vi "Delete Messages.vi"(8 "error in (no error)":errorcluster, 10 "Message":variant, 11 "Telegram Class in":refnum<class "Telegram Class.lvclass">) -> (0 "error out":errorcluster, 3 "Telegram Class out":refnum<class "Telegram Class.lvclass">)   [LabVIEW 2015, in "Telegram Library.lvlib" / "Telegram Class.lvclass"]
doc: "Created IvanLis by LabVIEW Portal\nProfile: http://labviewportal.org/memberlist.php?mode=viewprofile&u=987\neMail: IvanLisanov@gMail.com\nTelegram: https://t.me/IvanLis"
uses:
  Telegram Class.lvclass
  JSON Library/TypeDef/Delete Messages.ctl
  Telegram Class.lvclass/Telegram Class.ctl
  JSON Library/JSON Library.lvlib
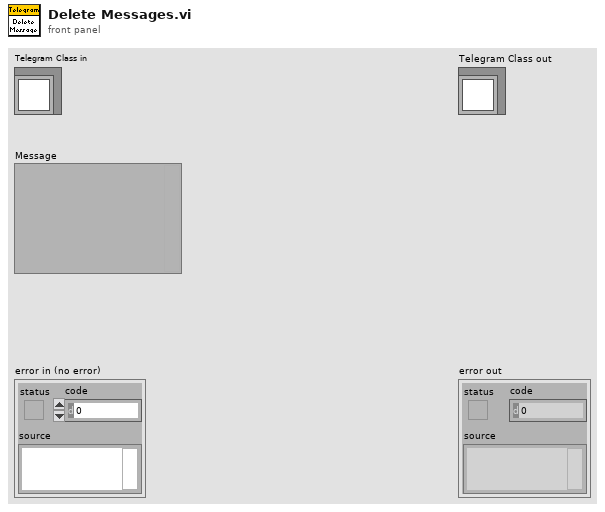
[diagram p1: front panel]
types:
  T1 = typedef "JSON Library.lvlib/Delete Messages.ctl" = cluster{"@type":string, "chat_id":i64, "message_ids":i64[]}
  T2 = typedef "Telegram Library.lvlib/Message.ctl" = cluster{"id":i64, "chat_id":i64, "sender_user_id":i64, "date UTC":timestamp, "content_text":string}
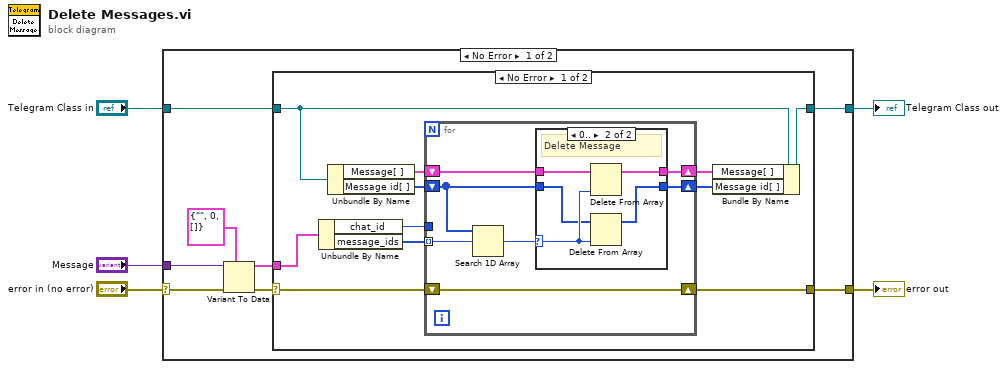
[diagram p0: block diagram]
diagram:
  n1 = case shown="No Error" "error in (no error)" {
    selector: "error in (no error)" -> [w13 w42]
    tunnel: [w8 w42] -> w4
    tunnel: [w6 w41] -> w2
    tunnel: "Telegram Class in" -> [w7 w41]
    tunnel: "Message" -> [w11 _]
    frame No Error {
      n2 = Variant To Data(error in=w13, type=T1 {"@type"="", "chat_id"=0, "message_ids"=[]} ("Message"), Variant=w11) -> (data=w10:T1, error out=w9:errorcluster)
      n3 = case shown="No Error" w9 {
        selector: w9 -> [w23 w40]
        tunnel: w10 -> [w19 _]
        tunnel: [w21 w40] -> w8
        tunnel: w7 -> [w18 w39]
        tunnel: [w16 w39] -> w6
        frame No Error {
          n4 = Unbundle By Name(w19) -> ("chat_id"=w22:i64, "message_ids"=w20:i64[])
          n5 = Unbundle By Name(w18) -> ("Message[ ]"=w24:T2[], "Message id[ ]"=w17:i64[])
          n6 = for {
            tunnel: w22 -> [_]
            tunnel: w20 -> [w31] mode=indexing
            shift-right: [w25] -> w21
            shift-left: w23 -> [w25]
            shift-right: [w27] -> w15
            shift-left: w24 -> [w28]
            shift-right: [w26] -> w14
            shift-left: w17 -> [w29]
            n7 = Search 1D Array(1D array=w29, element=w31) -> (index of element=w30:i32)  [unwired: 1 in]
            n8 = case shown="0.." w30 {
              selector: w30 -> [_ w36]
              tunnel: w29 -> [w32 w35]
              tunnel: w28 -> [w33 w38]
              tunnel: [w33 w37] -> w27
              tunnel: [w32 w34] -> w26
              frame ..-1 {
              }
              frame 0.. {
                # "Delete Message"
                n9 = Delete From Array(array=w38, index=w36) -> (array with subset deleted=w37:T2[])  [unwired: 1 in, 1 out]
                n10 = Delete From Array(array=w35, index=w36) -> (array with subset deleted=w34:i64[])  [unwired: 1 in, 1 out]
              }
            }
          }
          n11 = Bundle By Name(cluster=w18, "Message[ ]"=w15, "Message id[ ]"=w14) -> (w16:refnum<class "Telegram Class.lvclass">)
        }
        frame Error {
        }
      }
    }
    frame Error {
    }
  }
  "error out" <- w4
  "Telegram Class out" <- w2
